vi "Acquire microscope images.vi"() -> ()   [LabVIEW 2011]
doc: "Acquires sequences from the Andor iXon camera into Glimpse. \"Multi-mode\" means that the VI can be configured to sequentially acquire frames in multiple modes with different light sources and numbers of frames in each mode. Each mode is collected into a separate aquisition directory in Glimpse. Acquisition can be time-lapsed with a settable delay interval between cycles; the selected laser(s) are shuttered whilst not acquiring. The ixon setup acquisition.vi front panel is displayed so that the user can set the acquisition parameters before acquiring.\n\nThis is a Glimpse plug-in. To insure proper operation, you should have the source version of Glimpse running before loading this program. (The source version has an .llb extension, not a .exe one)."
uses:
  Glimpse core/GLIMPSE Globals.vi
  <vilib>/vision/Image Controls.llb/IMAQ Image.ctl
  glimpse core/Video acquisition state.ctl
  ixon camera/andor globals.vi
  Autofocus Globals.vi
  new-h-nu-ixon/stage globals.vi
  ixon1024/andor acquisition mode.ctl
  ixon1024/ixon readout settings.ctl
  h-nu-ixon/Laser type.ctt
  h-nu-ixon/Emission filters.ctl
panel:
  in  "# Fields across x":i8(slide)=3 min=1 max=10 step=1 scale=0.0..10.0
  in  "# Fields across y":i8(slide)=3 min=1 max=10 step=1 scale=0.0..10.0
  in  "Go? (F)":bool
  in  "Quit":bool
  in  "Preview?":bool
  in  "Delay after\nfilter change\n(ms)":u32
  in  "Scan fields options":T1(radio)
  in  "Scan Fields":bool
  in  "Max. cycles":i32=9999999
  in  "Cycle Interval (s)":dbl format="%_3f"
  in  "Camera Parameters":T4={"Exposure Time (sec)"=0.1, "EM CCD Gain"=230, "Readout Settings"={"Acquisition Mode"=enum."Frame Transfer Run till Abort", "Pixel Rate"=enum."EM CCD 5 Mhz 14 bits", "High Capacity?"=FALSE, "V Shift Speed (us/row)"=enum."0.9 (not reccommended)", "V Shift Amplitude"=enum."normal", "Preamp Gain"=enum."2.4", "Trigger Mode"=0}, "Image Size"={"H Bin"=1, "V Bin"=1, "Left"=1, "Top"=1, "Right"=512, "Bottom"=512}} {"Readout Settings"."Trigger Mode" items=["Internal", "External"]; "EM CCD Gain" scale=0.01..255.0; "Exposure Time (sec)" scale=0.001..10.0 scale format="%#_1g"}
  in  "Acquisition Protocol":T7(array[cluster]) {"Wait after frames (s)" format="%_3f"}
  # "Note:  In all panels, Ctrl-H displays the Context Help Window.  Hover mouse over panel icon or controls for context help."
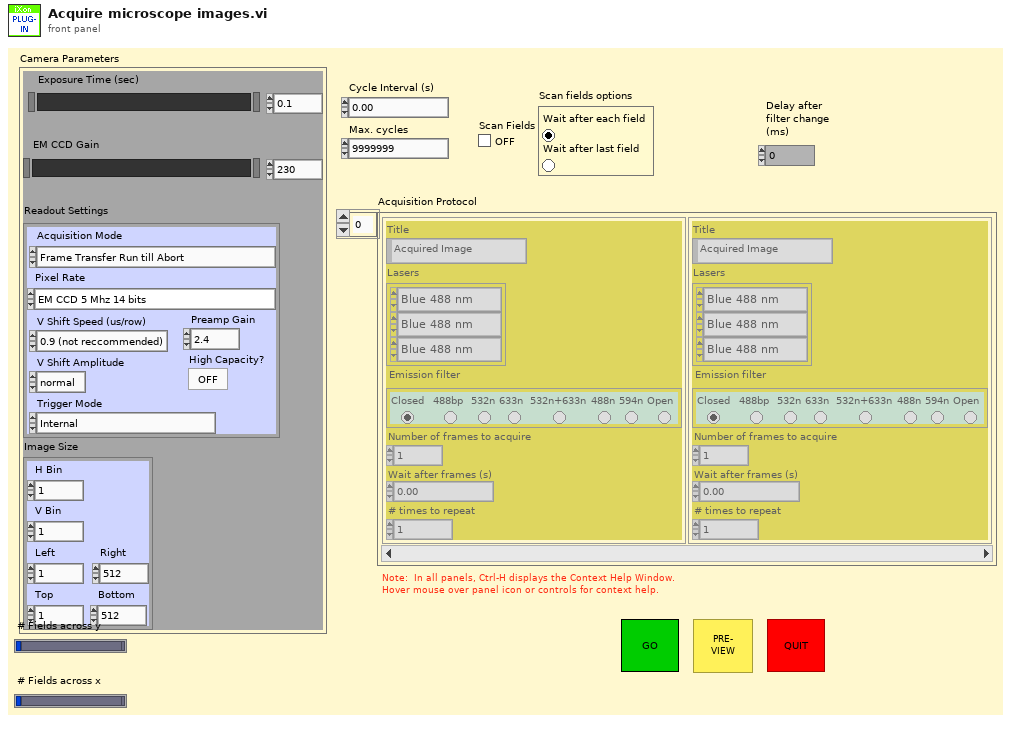
[diagram p1: front panel]
types:
  T1 = enum32{"Wait after each field", "Wait after last field"}
  T2 = typedef "ixon readout settings.ctl" = cluster{"Acquisition Mode":T3, "Pixel Rate":enum16{"EM CCD 10 Mhz 14 bits", "EM CCD 5 Mhz 14 bits", "EM CCD 3 Mhz 14 bits", "EM CCD 1 Mhz 16 bits", "Standard CCD 3 Mhz 14 bits", "Standard CCD 1 Mhz 16 bits"}, "High Capacity?":bool, "V Shift Speed (us/row)":enum16{"0.9 (not reccommended)", "1.7  (not reccommended)", "3.3  (not reccommended)", "6.5", "12.9"}, "V Shift Amplitude":enum16{"normal", "+1", "+2", "+3", "+4"}, "Preamp Gain":enum16{"1.0", "2.4", "5.0"}, "Trigger Mode":u32}
  T3 = typedef "andor acquisition mode.ctl" = enum16{"(do not use)", "Single Scan", "Accumulate", "Kinetics", "Fast Kinetics", "Kinetics Run till Abort", "Frame Transfer", "Frame Transfer Run till Abort", "(do not use) ", "Time Delayed Integration"}
  T4 = cluster{"Exposure Time (sec)":sgl, "EM CCD Gain":u8, "Readout Settings":T2, "Image Size":cluster{"H Bin":i32, "V Bin":i32, "Left":i32, "Top":i32, "Right":i32, "Bottom":i32}}
  T5 = typedef "Laser type.ctt" = enum16{"Blue 488 nm", "Green 532 nm", "Orange 594 nm", "Red 633 nm", "IR 780"}
  T6 = typedef "Emission filters.ctl" = enum32{" Closed ", "488bp ", "532n", "633n ", "532n+633n", "488n", "594n", "Open"}
  T7 = cluster{"Title":string, "Lasers":T5[], "Emission filter":T6, "Number of frames to acquire":i32, "Wait after frames (s)":dbl, "# times to repeat":i32}[]
  T8 = typedef "Video acquisition state.ctl" = cluster{"Pixel depth":enum32{"8 bits", "16 bits", "Float", "Complex", "RGB Chunky", "Compressed"}, "Width":dbl, "Height":dbl, "Buffer":T9, "Frames Acquired":u32, "Time of 1st frame":dbl, "TTB element zero":u32, "File Offsets Array":cluster{"offset":i32, "file number":u8}[], "TTB Array":u32[], "Sum Image (for averaging)":T9}
  T9 = typedef "IMAQ Image.ctl" = refnum<image>
  T10 = enum32{"None", "Manual", "Auto - Image analysis", "Auto - Retro-reflection"}
  T11 = cluster{"H Bin":i32, "V Bin":i32, "Left":i32, "Top":i32, "Right":i32, "Bottom":i32}
  T12 = typedef "Video acquisition state.ctl" = cluster{"Pixel depth":enum32{"8 bits", "16 bits", "Float", "Complex", "RGB Chunky", "Compressed"}, "Width":dbl, "Height":dbl, "Buffer":T9, "Frames Acquired":u32, "Time of 1st frame":dbl, "TTB element zero":u32, "File Offsets Array":T13, "TTB Array":u32[], "Sum Image (for averaging)":T9, "Time at end of last acquisition (ms)":u32, "Filter array":u16[], "Flow rate array":dbl[], "Temperature array":dbl[], "Field array":u16[], "Lasers array":u16[][], "Stage xyz array":dbl[][]}
  T13 = typedef "Offset table.ctl" = cluster{"offset":T14, "file number":T15}[]
  T14 = typedef "Offset.ctl" = i32
  T15 = typedef "file number.ctl" = u8
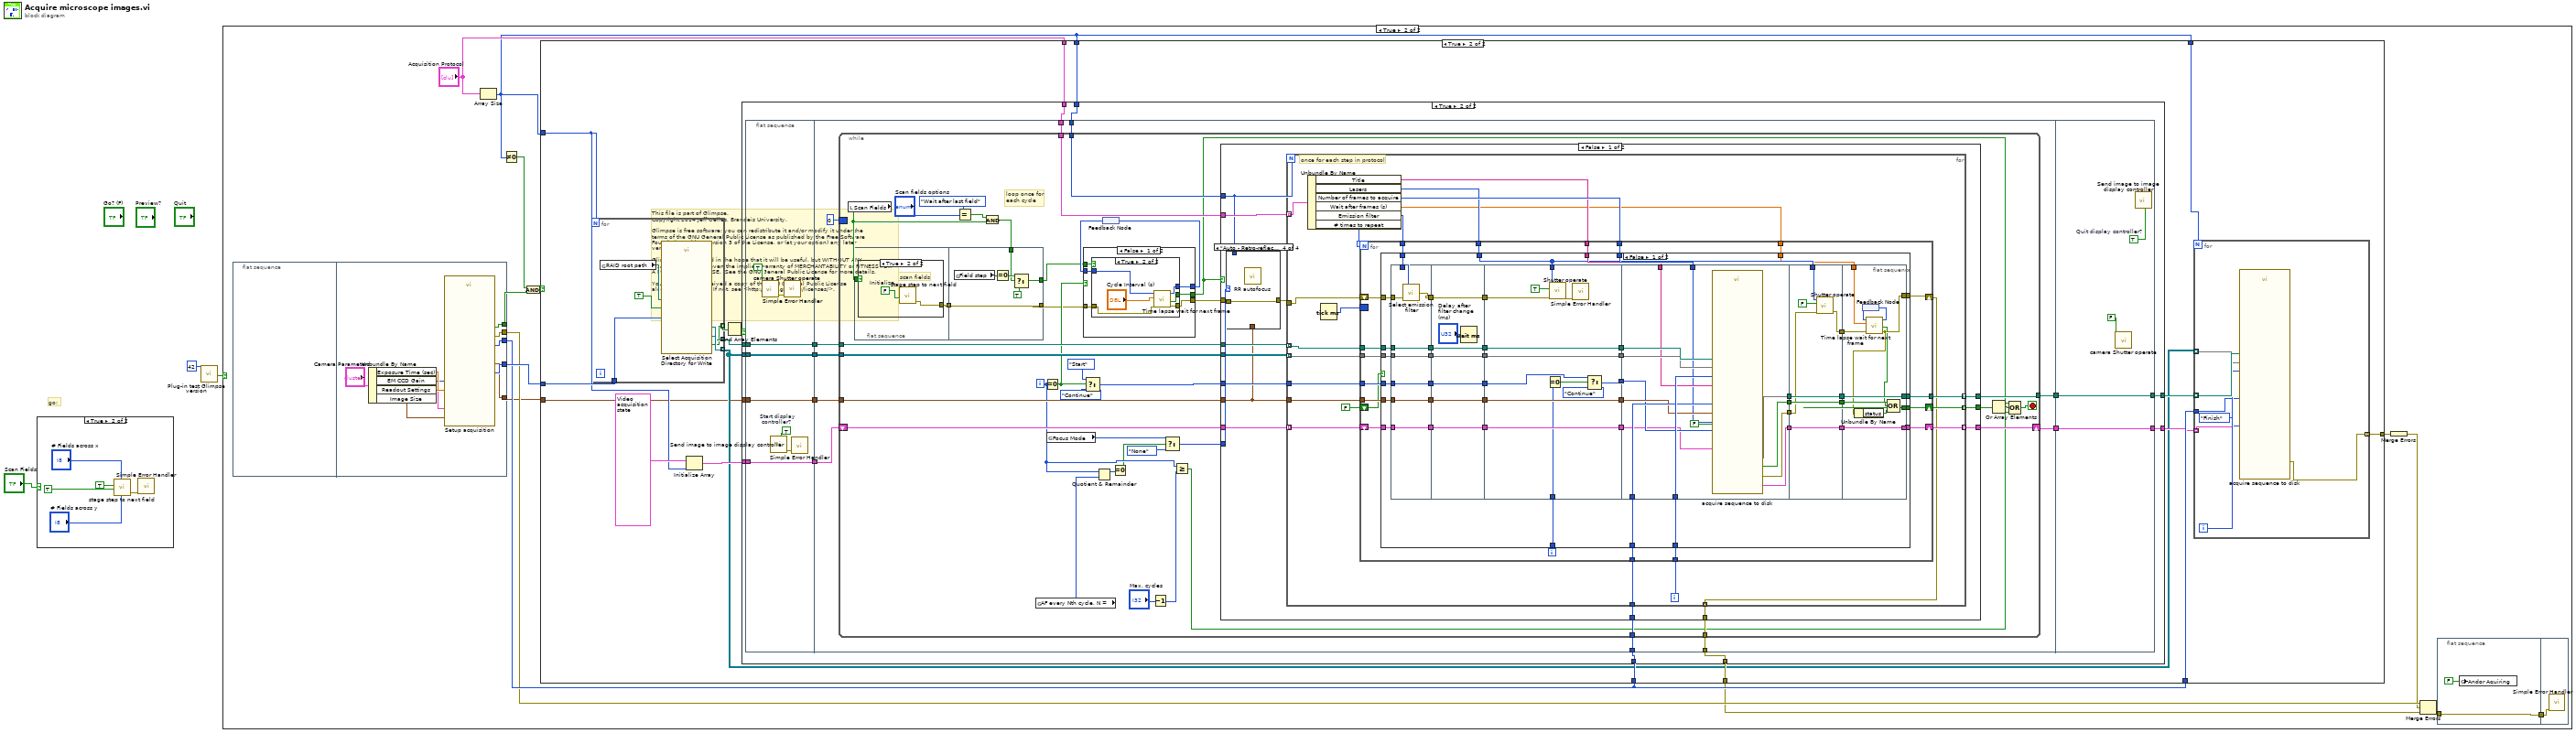
[diagram p0: block diagram]
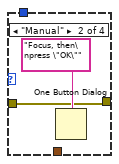
[diagram p7: hidden frame]
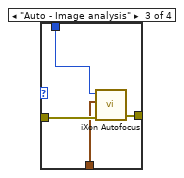
[diagram p8: hidden frame]
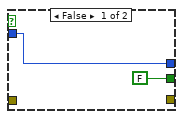
[diagram p12: hidden frame]
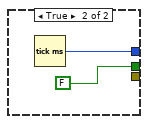
[diagram p13: hidden frame]
diagram:
  # "This file is part of Glimpse. \nCopyright 2014 Jeff Gelles, Brandeis University.    \n\nGlimpse is free software: you can redistribute it and/or modify it under the \nterms of the GNU General Public License as published by the Free Software \nFoundation, either version 3 of the License, or (at your option) any later \nversion.\n\nGlimpse is distributed in the hope that it will be useful, but WITHOUT ANY \nWARRANTY; without even the implied warranty of MERCHANTABILITY or FITNESS FOR \nA PARTICULAR PURPOSE.  See the GNU General Public License for more details.\n\nYou should have received a copy of the GNU General Public License\nalong with Glimpse.  If not, see <http://www.gnu.org/licenses/>."
  # "go:"
  n1 = case shown="True" "Scan Fields" {
    frame False {
    }
    frame True {
      n2 = call "stage step to next field.vi"("# Fields across x"="# Fields across x", "Go"=TRUE, "Initialize"=TRUE, "# Fields across y"="# Fields across y") -> ("error out"=w8:errorcluster)  [unwired: 4 in]
      n3 = call <vilib>:"Simple Error Handler.vi"("error in (no error)"=w8) -> ()  [unwired: 1 in, 8 out]
    }
  }
  n4 = call "Plug-in test Glimpse version.vi"("Minimum version required"=42) -> ("OK?"=w3:bool)  [unwired: 6 out]
  n5 = case shown="True" w3 {
    frame False {
    }
    frame True {
      n6 = flat-sequence {
        tunnel: [w35] -> w22
        tunnel: [w34] -> w21
        tunnel: [w33] -> w20
        tunnel: [w31] -> w14
        tunnel: [w26] -> w11
        frame #0 {
        }
        frame #1 {
          n7 = Unbundle By Name("Camera Parameters") -> ("Exposure Time (sec)"=w30:sgl, "EM CCD Gain"=w29:u8, "Readout Settings"=w28:T2, "Image Size"=w27:T11)
          n8 = call "Setup acquisition.vi"("Exposure Time (sec)"=w30, "EM CCD Gain"=w29, "Image Size"=w27, "Readout Settings"=w28) -> ("Image Size Out"=w26:T11, "Continue with acq?"=w31:bool, "Number of acquisition files"=w35:i8, "Frames per acquisition file"=w34:u32, "Error Out (no error)"=w33:errorcluster)  [unwired: 4 in, 7 out]
        }
      }
      n9 = Array Size(array="Acquisition Protocol") -> (size(s)=w13:i32)
      n10 = Not Equal To 0?(x=w13) -> (x != 0?=w12:bool)
      n11 = And(x=w12, y=w14) -> (x .and. y?=w15:bool)
      n12 = case shown="True" w15 {
        tunnel: w22 -> [_ w52]
        tunnel: w21 -> [_ w51]
        tunnel: w21 -> [_ w50]
        tunnel: [_ w49] -> w18
        tunnel: [_ w48] -> w19
        tunnel: w13 -> [_ w37]
        tunnel: w13 -> [_ w43]
        tunnel: w13 -> [_ w40]
        tunnel: "Acquisition Protocol" -> [_ w38]
        tunnel: w11 -> [_ w36]
        frame False {
        }
        frame True {
          n13 = for {
            N: w37 -> [_]
            tunnel: [w342] -> w39 mode=indexing
            tunnel: [w341] -> w44 mode=indexing
            tunnel: [w340] -> w53 mode=indexing
            tunnel: w52 -> [w339]
            n14 = global read "GLIMPSE Globals.vi" "RAID root path"() -> (w344:path)
            n15 = call "Select Acquisition Directory for Write.vi"("Autostart?"=TRUE, "Acquisition directory root path"=w344, "Number of acquisition files"=w339) -> ("Acquisition files refnums array"=w342:refnum<file>[], "OK?"=w340:bool, "Directory Path Out"=w341:path)  [unwired: 10 out]
          }
          n16 = Initialize Array(T8 {"Pixel depth"=enum."8 bits", "Width"=0.0, "Height"=0.0, "Buffer"=refnum, "Frames Acquired"=0, "Time of 1st frame"=0.0, "TTB element zero"=0, "File Offsets Array"=[], "TTB Array"=[], "Sum Image (for averaging)"=refnum} ("State Out"), w37) -> (w41:T8[])
          n17 = And Array Elements(Boolean array=w53) -> (logical AND=w45:bool)
          n18 = case shown="True" w45 {
            tunnel: [w62 w78] -> w47
            tunnel: w39 -> [_ w77]
            tunnel: w51 -> [_ w76]
            tunnel: [w61 w75] -> w46
            tunnel: [_ w74] -> w49
            tunnel: w44 -> [w62 w73]
            tunnel: w43 -> [_ w72]
            tunnel: w41 -> [w61 w71]
            tunnel: w38 -> [_ w70]
            tunnel: w36 -> [_ w64]
            frame False {
            }
            frame True {
              n19 = flat-sequence {
                tunnel: w71 -> [w84]
                tunnel: w73 -> [w85]
                tunnel: w77 -> [w86]
                tunnel: [w86] -> w69
                tunnel: [w85] -> w68
                tunnel: [w84] -> w67
                tunnel: w64 -> [w82]
                tunnel: [w82] -> w63
                tunnel: w76 -> [w95]
                tunnel: [w93] -> w74
                tunnel: w72 -> [w91]
                tunnel: w70 -> [w89]
                tunnel: w69 -> [w96]
                tunnel: w68 -> [w92]
                tunnel: w67 -> [w90]
                tunnel: [w97] -> w66
                tunnel: [w94] -> w65
                tunnel: w63 -> [w88]
                tunnel: [w337] -> w75
                tunnel: [w338] -> w78
                tunnel: w66 -> [w338]
                tunnel: w65 -> [w337]
                frame #0 {
                  w81 = TRUE  # Start display  controller?
                  n20 = call "camera Shutter operate.vi"("Open?"=TRUE) -> ("error out"=w79:errorcluster)  [unwired: 1 in, 6 out]
                  n21 = call "Send image to image display controller.vi"("Start display controller?"=w81) -> ("error out"=w80:errorcluster)  [unwired: 6 in, 3 out]
                  n22 = call <vilib>:"Simple Error Handler.vi"("error in (no error)"=w79) -> ()  [unwired: 1 in, 8 out]
                  n23 = call <vilib>:"Simple Error Handler.vi"("error in (no error)"=w80) -> ()  [unwired: 1 in, 8 out]
                }
                frame #1 {
                  n24 = while {
                    tunnel: [w136] -> w97
                    tunnel: w96 -> [w135]
                    tunnel: w95 -> [w134]
                    shift-right: [w132] -> w94
                    shift-left: w90 -> [w133]
                    tunnel: [w131] -> w93
                    tunnel: w92 -> [w130]
                    tunnel: w91 -> [w118]
                    tunnel: w89 -> [w124]
                    tunnel: w88 -> [w119]
                    border: u32 0 -> [_]
                    i -> [w115]
                    stop <- w122 stop-if-true
                    # "loop once for\neach cycle"
                    n25 = local read "Scan Fields"() -> (w104:bool)
                    n26 = flat-sequence {
                      tunnel: w104 -> [w310]
                      tunnel: [w309] -> w105
                      tunnel: [w318] -> w110
                      tunnel: w105 -> [w318]
                      tunnel: w102 -> [w314]
                      tunnel: [w313] -> w103
                      frame #0 {
                        n27 = case shown="True" w310 {
                          tunnel: [_ w311] -> w309
                          frame False {
                          }
                          frame True {
                            w312 = FALSE  # Initialize
                            # "scan fields"
                            n28 = call "stage step to next field.vi"("Initialize"=w312) -> ("error out"=w311:errorcluster)  [unwired: 2 in, 4 out]
                          }
                        }
                      }
                      frame #1 {
                        n29 = global read "stage globals.vi" "Field step"() -> (w315:i16)
                        n30 = Equal To 0?(x=w315) -> (x = 0?=w316:bool)
                        n31 = Select(t=w316, s=w314, f=TRUE) -> (s? t:f=w313:bool)
                      }
                    }
                    n32 = Equal?(x="Scan fields options", y=T1."Wait after last field") -> (x = y?=w101:bool)
                    n33 = And(x=w101, y=w104) -> (x .and. y?=w102:bool)
                    n34 = global read "Autofocus Globals.vi" "AF every Nth cycle, N ="() -> (w117:u8)
                    n35 = Equal To 0?(x=w115) -> (x = 0?=w123:bool)
                    n36 = global read "Autofocus Globals.vi" "Focus Mode"() -> (w108:T10)
                    n37 = Select(t=enum16{"Start", "Continue", "Finish"}."Start" ("Operation"), s=w123, f=enum16{"Start", "Continue", "Finish"}."Continue" ("Operation")) -> (s? t:f=w127:enum16{"Start", "Continue", "Finish"})
                    n38 = Quotient & Remainder(x=w115, y=w117) -> (x-y*floor(x/y)=w116:i32)  [unwired: 1 out]
                    n39 = feedback #1() -> (w120:u32)
                    n40 = case shown="False" w123 {
                      tunnel: [w324 w334] -> w121
                      tunnel: [w323 FALSE] -> w98
                      tunnel: w120 -> [w322 _]
                      tunnel: [w321 _] -> w111
                      tunnel: w103 -> [w320 _]
                      tunnel: w110 -> [w319 _]
                      frame False {
                        n41 = case shown="True" w320 {
                          tunnel: [w326 w332] -> w324
                          tunnel: [FALSE ("Stopped?") w331] -> w323
                          tunnel: w322 -> [w326 w330]
                          tunnel: [_ w328] -> w321
                          tunnel: w319 -> [_ w327]
                          frame False {
                          }
                          frame True {
                            n42 = call "Time lapse wait for next frame.vi"("error in (no error)"=w327, "Frame Interval (s)"="Cycle Interval (s)", "Time of last frame in"=w330) -> ("error out"=w328:errorcluster, "Stopped?"=w331:bool, "Time of this frame out (ms)"=w332:u32)  [unwired: 4 out]
                          }
                        }
                      }
                      frame True {
                        n43 = Tick Count (ms)() -> (millisecond timer value=w334:u32)
                      }
                    }
                    n44 = feedback-in #1(w121) -> ()
                    n45 = Equal To 0?(x=w116) -> (x = 0?=w109:bool)
                    n46 = Decrement(x="Max. cycles") -> (x-1=w112:i32)
                    n47 = Select(t=w108, s=w109, f=T10."None") -> (s? t:f=w106:T10)
                    n48 = Greater Or Equal?(x=w115, y=w112) -> (x >= y?=w113:bool)
                    n49 = case shown="False" w98 {
                      tunnel: [w151 w308] -> w136
                      tunnel: w135 -> [w150 _]
                      tunnel: w134 -> [w149 _]
                      tunnel: w133 -> [w148 w307]
                      tunnel: [w147 w307] -> w132
                      tunnel: [w146 _] -> w131
                      tunnel: w130 -> [w145 w308]
                      tunnel: w127 -> [w144 _]
                      tunnel: [w143 _] -> w126
                      tunnel: w124 -> [w142 _]
                      tunnel: w119 -> [w140 _]
                      tunnel: w118 -> [w139 _]
                      tunnel: w111 -> [w138 _]
                      tunnel: w106 -> [w137 _]
                      frame False {
                        n50 = case shown="\"Auto - Retro-reflection\"" w137 {
                          tunnel: w138 -> [w152 w153 w158 w159]
                          tunnel: [w152 w153 w157 w159] -> w141
                          tunnel: w140 -> [_ _ w156 _]
                          tunnel: w139 -> [_ _ w155 _]
                          frame "None", Default {
                          }
                          frame "Manual" {
                            n51 = One Button Dialog(message="Focus, then\npress \"OK\"") -> ()  [unwired: 2 out]
                          }
                          frame "Auto - Image analysis" {
                            n52 = call "iXon Autofocus.vi"("error in"=w158, "Image Size"=w156, "Display Window Number"=w155) -> ("error out"=w157:errorcluster)  [unwired: 2 in, 6 out]
                          }
                          frame "Auto - Retro-reflection" {
                            n53 = call "RR autofocus.vi"() -> ()  [unwired: 2 out]
                          }
                        }
                        n54 = for {
                          N: w139 -> [_]
                          tunnel: [w180] -> w151 mode=indexing
                          tunnel: w150 -> [w179] mode=indexing
                          tunnel: w149 -> [w178]
                          tunnel: w148 -> [w172] mode=indexing
                          tunnel: [w177] -> w147 mode=indexing
                          tunnel: [w176] -> w143 mode=indexing
                          tunnel: [w175] -> w146 mode=indexing
                          tunnel: w145 -> [w174] mode=indexing
                          tunnel: w144 -> [w173]
                          tunnel: w142 -> [w171] mode=indexing
                          tunnel: w141 -> [w167]
                          tunnel: w140 -> [w166]
                          i -> [w169]
                          # "once for each step in protocol"
                          n55 = Unbundle By Name(w171) -> ("Title"=w168:string, "Lasers"=w165:T5[], "Number of frames to acquire"=w170:i32, "Wait after frames (s)"=w163:dbl, "Emission filter"=w160:T6, "# times to repeat"=w161:i32)
                          n56 = Tick Count (ms)() -> (millisecond timer value=w164:u32)
                          n57 = for {
                            N: w161 -> [_]
                            tunnel: [w199] -> w180
                            tunnel: w179 -> [w198]
                            tunnel: w178 -> [w197]
                            tunnel: w174 -> [w193]
                            tunnel: w173 -> [w192]
                            tunnel: w170 -> [w190]
                            tunnel: w169 -> [w189]
                            tunnel: w168 -> [w188]
                            tunnel: w166 -> [w186]
                            tunnel: w165 -> [w185]
                            shift-right: [w196] -> w177
                            shift-left: w172 -> [w191]
                            border: w164 -> [_]
                            tunnel: w163 -> [w184]
                            shift-right: [w195] -> w176
                            shift-left: FALSE -> [w183]
                            shift-right: [w194] -> w175
                            shift-left: w167 -> [w187]
                            tunnel: w160 -> [w181]
                            i -> [w182]
                            n58 = case shown="False" w183 {
                              selector: w183 -> [_ w305]
                              tunnel: [w229 w306] -> w199
                              tunnel: w198 -> [w228 _]
                              tunnel: w197 -> [w227 _]
                              tunnel: [w226 w304] -> w196
                              tunnel: [w225 w305] -> w195
                              tunnel: [w224 w303] -> w194
                              tunnel: w193 -> [w223 w306]
                              tunnel: w192 -> [w222 _]
                              tunnel: w191 -> [w221 w304]
                              tunnel: w190 -> [w220 _]
                              tunnel: w189 -> [w219 _]
                              tunnel: w188 -> [w218 _]
                              tunnel: w187 -> [w217 w303]
                              tunnel: w186 -> [w216 _]
                              tunnel: w185 -> [w215 _]
                              tunnel: w184 -> [w214 _]
                              tunnel: w182 -> [w213 _]
                              tunnel: w181 -> [w212 _]
                              frame False {
                                n59 = flat-sequence {
                                tunnel: w216 -> [w246]
                                tunnel: w217 -> [w244]
                                tunnel: w221 -> [w247]
                                tunnel: w222 -> [w248]
                                tunnel: w223 -> [w249]
                                tunnel: w228 -> [w250]
                                tunnel: [w250] -> w211
                                tunnel: [w249] -> w209
                                tunnel: [w248] -> w207
                                tunnel: [w247] -> w205
                                tunnel: [w243] -> w203
                                tunnel: [w246] -> w201
                                tunnel: w212 -> [w245]
                                tunnel: w211 -> [w257]
                                tunnel: [w257] -> w210
                                tunnel: w209 -> [w256]
                                tunnel: [w256] -> w208
                                tunnel: w207 -> [w255]
                                tunnel: [w255] -> w206
                                tunnel: w205 -> [w254]
                                tunnel: [w254] -> w204
                                tunnel: w203 -> [w253]
                                tunnel: [w253] -> w202
                                tunnel: w201 -> [w252]
                                tunnel: [w252] -> w200
                                tunnel: [w266] -> w242
                                tunnel: [w270] -> w241
                                tunnel: w215 -> [w267]
                                tunnel: [w259] -> w240
                                tunnel: [w265] -> w239
                                tunnel: [w264] -> w238
                                tunnel: w213 -> [w261]
                                tunnel: w210 -> [w270]
                                tunnel: w208 -> [w266]
                                tunnel: w206 -> [w260]
                                tunnel: w204 -> [w265]
                                tunnel: w202 -> [w258]
                                tunnel: w200 -> [w264]
                                tunnel: w242 -> [w284]
                                tunnel: w241 -> [w283]
                                tunnel: [w272] -> w237
                                tunnel: [w271] -> w236
                                tunnel: [w273] -> w235
                                tunnel: w227 -> [w280]
                                tunnel: [w274] -> w234
                                tunnel: w240 -> [w277]
                                tunnel: w239 -> [w275]
                                tunnel: w220 -> [w278]
                                tunnel: w219 -> [w282]
                                tunnel: w218 -> [w281]
                                tunnel: w238 -> [w279]
                                tunnel: w237 -> [w291]
                                tunnel: [w291] -> w233
                                tunnel: w236 -> [w290]
                                tunnel: [w290] -> w232
                                tunnel: w235 -> [w286]
                                tunnel: w234 -> [w289]
                                tunnel: [w289] -> w231
                                tunnel: w215 -> [w287]
                                tunnel: [w285] -> w230
                                tunnel: [w301] -> w229
                                tunnel: [w302] -> w226
                                tunnel: w233 -> [w302]
                                tunnel: w232 -> [w301]
                                tunnel: w231 -> [w299]
                                tunnel: [w298] -> w225
                                tunnel: [w293] -> w224
                                tunnel: w214 -> [w295]
                                tunnel: w230 -> [w294]
                                frame #0 {
                                n60 = call "Select emission filter.vi"("error in"=w244, "Emission filter"=w245) -> ("error out"=w243:errorcluster)
                                }
                                frame #1 {
                                n61 = Wait (ms)(milliseconds to wait="Delay after\nfilter change\n(ms)") -> ()  [unwired: 1 out]
                                }
                                frame #2 {
                                n62 = Equal To 0?(x=w261) -> (x = 0?=w262:bool)
                                n63 = call "Shutter operate.vi"("Shutters"=w267, 2:TRUE ("Data to Write"), "error in"=w258) -> ("error out"=w268:errorcluster)  [unwired: 5 out]
                                n64 = call <vilib>:"Simple Error Handler.vi"("error in (no error)"=w268) -> ()  [unwired: 1 in, 8 out]
                                n65 = Select(t=w260, s=w262, f=enum16{"Start", "Continue", "Finish"}."Continue" ("Operation")) -> (s? t:f=w259:enum16{"Start", "Continue", "Finish"})
                                }
                                frame #3 {
                                n66 = call "acquire sequence to disk.vi"("Image Size"=w279, "State In"=w275, "Frames per acquisition file"=w280, "Sequence files handle"=w284, "Description Info"=w283, "Pressing stop automatically runs finish?"=FALSE, "Display Window Title"=w281, "Operation"=w277, "Display Window Number"=w282, "Number of frames to acquire"=w278) -> ("Done?"=w274:bool, "State Out"=w272:T12, 17:w271, "error out"=w273:errorcluster)  [unwired: 1 in, 5 out]
                                }
                                frame #4 {
                                n67 = call "Shutter operate.vi"("Shutters"=w287, 2:FALSE ("Data to Write"), "error in"=w286) -> ("error out"=w285:errorcluster)  [unwired: 5 out]
                                }
                                frame #5 {
                                n68 = feedback #2() -> (w296:u32)
                                n69 = call "Time lapse wait for next frame.vi"("error in (no error)"=w294, "Frame Interval (s)"=w295, "Time of last frame in"=w296) -> ("error out"=w293:errorcluster, "Stopped?"=w292:bool, "Time of this frame out (ms)"=w297:u32)  [unwired: 4 out]
                                n70 = Unbundle By Name(w293) -> ("status"=w300:bool)
                                n71 = feedback-in #2(w297) -> ()
                                n72 = Compound Arithmetic op=OR(w292, w299, w300) -> (w298:bool)
                                }
                                }
                              }
                              frame True {
                              }
                            }
                          }
                        }
                      }
                      frame True {
                      }
                    }
                    n73 = Or Array Elements(Boolean array=w126) -> (logical OR=w125:bool)
                    n74 = Compound Arithmetic op=OR(w98, w125, w113) -> (w122:bool)
                  }
                }
                frame #2 {
                  w336 = TRUE  # Quit display controller?
                  n75 = call "camera Shutter operate.vi"("Open?"=FALSE) -> ()  [unwired: 1 in, 7 out]
                  n76 = call "Send image to image display controller.vi"("Quit display controller?"=w336) -> ()  [unwired: 6 in, 4 out]
                }
              }
            }
          }
          n77 = for {
            N: w40 -> [_]
            tunnel: w50 -> [w57]
            tunnel: [w54] -> w48 mode=indexing
            tunnel: w47 -> [w60] mode=indexing
            tunnel: w46 -> [w55] mode=indexing
            tunnel: w39 -> [w59] mode=indexing
            i -> [w58]
            n78 = call "acquire sequence to disk.vi"("State In"=w55, "Frames per acquisition file"=w57, "Sequence files handle"=w60, "Description Info"=w59, "Operation"=enum16{"Start", "Continue", "Finish"}."Finish", "Display Window Number"=w58) -> ("error out"=w54:errorcluster)  [unwired: 6 in, 7 out]
          }
        }
      }
      n79 = Merge Errors(w19) -> (w17:errorcluster)
      n80 = Merge Errors(w20, w17, w18) -> (w10:errorcluster)
      n81 = flat-sequence {
        tunnel: w10 -> [w23]
        tunnel: [w23] -> w9
        tunnel: w9 -> [w25]
        frame #0 {
          n82 = global write "andor globals.vi" "Andor Aquiring"(FALSE ("Andor Aquiring")) -> ()
        }
        frame #1 {
          n83 = call <vilib>:"Simple Error Handler.vi"("error in (no error)"=w25) -> ()  [unwired: 1 in, 8 out]
        }
      }
    }
  }
